vi "sub_Check_Rx_Packet_Validity.vi"(6 "PSK Init Parameters":T2, 9 "Packet Parameters":T3, 10 "Input Bit Stream":cluster{"bit stream ":i8[][], "Enable?":bool}) -> (3 "Output Bit Stream":T1)   [LabVIEW 2014]
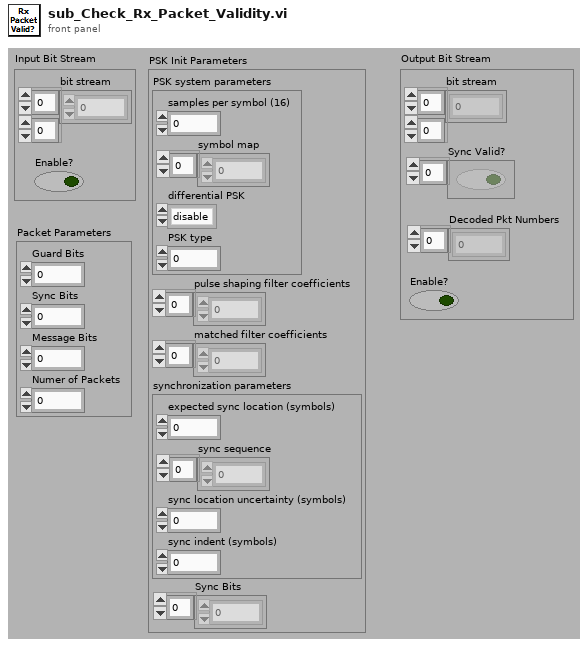
[diagram p1: front panel]
types:
  T1 = cluster{"bit stream ":i8[][], "Sync Valid?":bool[], "Decoded Pkt Numbers":u32[], "Enable?":bool}
  T2 = cluster{"PSK system parameters":cluster{"samples per symbol (16)":i32, "symbol map":cdb[], "differential PSK":enum16{"disable", "enable"}, "PSK type":u16}, "pulse shaping filter coefficients":dbl[], "matched filter coefficients":dbl[], "synchronization parameters":cluster{"expected sync location (symbols)":i32, "sync sequence":cdb[], "sync location uncertainty (symbols)":i32, "sync indent (symbols)":i32}, "Sync Bits":i8[]}
  T3 = cluster{"Guard Bits ":i32, "Sync Bits":i32, "Message Bits":i32, "Numer of Packets":i32}
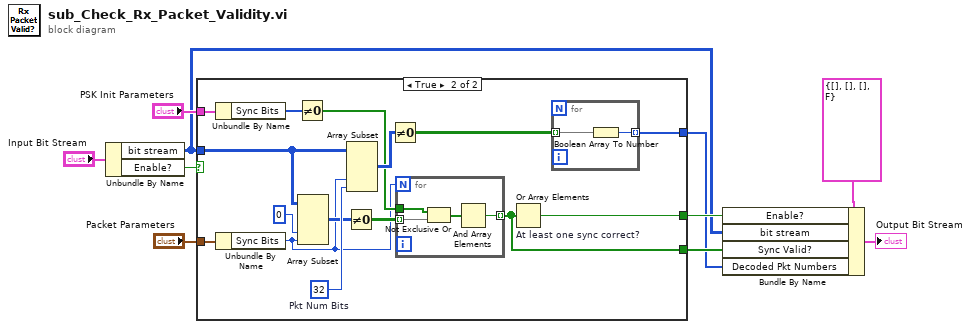
[diagram p0: block diagram]
diagram:
  n1 = Unbundle By Name("Input Bit Stream") -> ("bit stream"=w5:i8[][], "Enable?"=w8:bool)
  n2 = case shown="True" w8 {
    selector: w8 -> [w11 _]
    tunnel: w5 -> [_ w21]
    tunnel: "Packet Parameters" -> [_ w26]
    tunnel: "PSK Init Parameters" -> [_ w14]
    tunnel: [_ w20] -> w4
    tunnel: [_ w22] -> w3
    tunnel: [w11 w19] -> w6
    frame False {
    }
    frame True {
      w24 = 32  # Pkt Num Bits
      n3 = Unbundle By Name(w14) -> ("Sync Bits"=w13:i8[])
      n4 = Unbundle By Name(w26) -> ("Sync Bits"=w12:i32)
      n5 = Not Equal To 0?(x=w13) -> (x != 0?=w18:bool[])
      n6 = Array Subset(array=w21, index (col)=0 ("index"), length (col)=w12) -> (w16:i8[][])  [unwired: 2 in]
      n7 = Not Equal To 0?(x=w16) -> (x != 0?=w15:bool[][])
      n8 = Array Subset(array=w21, index (col)=w12, length (col)=w24) -> (w23:i8[][])  [unwired: 2 in]
      n9 = Not Equal To 0?(x=w23) -> (x != 0?=w17:bool[][])
      n10 = for {
        N: w12 -> [_]
        tunnel: [w30] -> w20 mode=indexing
        tunnel: w18 -> [w28]
        tunnel: w15 -> [w27] mode=indexing
        n11 = Not Exclusive Or(1:w27, 2:w28) -> (0:w29:bool[])
        n12 = And Array Elements(Boolean array=w29) -> (logical AND=w30:bool)
      }
      n13 = Or Array Elements "At least one sync correct?"(Boolean array=w20) -> (logical OR=w19:bool)
      n14 = for {
        tunnel: [w32] -> w22 mode=indexing
        tunnel: w17 -> [w31] mode=indexing
        n15 = Boolean Array To Number(Boolean array=w31) -> (number=w32:u32)
      }
    }
  }
  n16 = Bundle By Name(cluster=T1 {"bit stream "=[], "Sync Valid?"=[], "Decoded Pkt Numbers"=[], "Enable?"=FALSE} ("Output Bit Stream"), "Enable?"=w6, "bit stream"=w5, "Sync Valid?"=w4, "Decoded Pkt Numbers"=w3) -> (→"Output Bit Stream":T1)
